vi "Execute SQL Statement.vi"(8 "error in (no error)":errorcluster, 10 "SQL string":string, 11 "Data.PGQL in":refnum<class "LV-Data.PGSQL.lvclass">) -> (0 "error out":errorcluster, 1 "Result":string[][](array[string]), 3 "Data.PGSQL out":refnum<class "LV-Data.PGSQL.lvclass">)   [LabVIEW 2019, in "LV-Data.PGSQL.lvclass"]
uses:
  LV-Data.PGSQL.lvclass
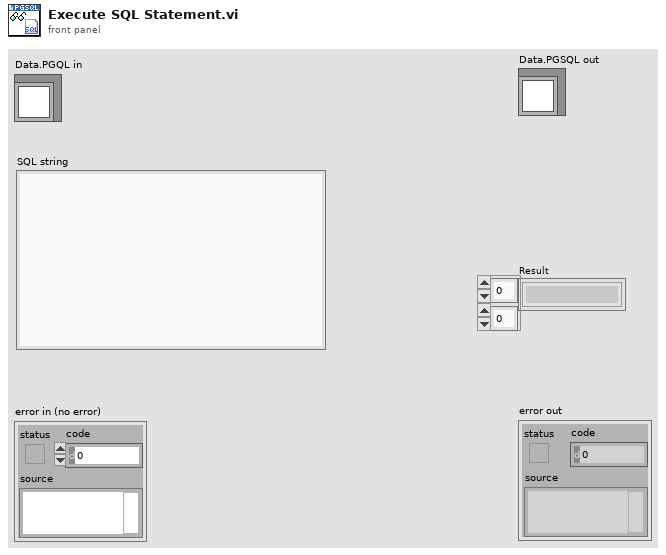
[diagram p1: front panel]
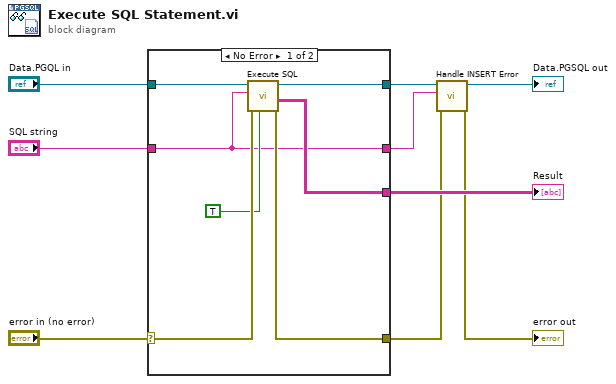
[diagram p0: block diagram]
diagram:
  n1 = case shown="No Error" "error in (no error)" {
    selector: "error in (no error)" -> [w13 w18]
    tunnel: "Data.PGQL in" -> [w16 w19]
    tunnel: "SQL string" -> [w10 w17]
    tunnel: [w15 w18] -> w2
    tunnel: [w14 w19] -> w4
    tunnel: [w11 _] -> w8
    tunnel: [w10 w17] -> w5
    frame No Error {
      n2 = call "Execute SQL.vi"("Result?"=TRUE, "error in"=w13, "SQL"=w10, "LV-Data.PGSQL"=w16) -> ("error out"=w15:errorcluster, "Result"=w11:string[][], "LV-Data.PGSQL out"=w14:refnum<class "LV-Data.PGSQL.lvclass">)  [unwired: 4 in, 1 out]
    }
    frame Error {
    }
  }
  "Result" <- w8
  n3 = call "Handle INSERT Error.vi"("error in (no error)"=w2, "SQL"=w5, "Database.PG"=w4) -> ("error out"=→"error out":errorcluster, "Database.PG out"=→"Data.PGSQL out":refnum<class "LV-Data.PGSQL.lvclass">)  [unwired: 6 in, 1 out]
